vi "Set Calibrator Range.vi"(8 "error in (no error)":errorcluster, 10 "Calibrator Range (0: 10 mV)":u32(ring) items=["10 mV", "25 mV", "100 mV", "250 mV", "1 V", "2.5 V", "Res 50 ohm", "Res 1 Mohm", "Capacitance", "DC", "AC"], 11 "VISA resource name":refnum<visa-resource-name>) -> (0 "error out":errorcluster, 3 "VISA resource name out":refnum<visa-resource-name>)   [LabVIEW 2011, in "Fluke 5XXX Series Multicalibrators.lvlib"]
doc: "This VI programs the instrument range in Pulse, Impedance & Capacitance Measurement and Overload scope modes.\n\nNote:\n\nThis VI is available only for instrument models 5500A and 5520A with oscilloscope option SC600 (SC1100)."
uses:
  Fluke 5XXX Series Multicalibrators.lvlib
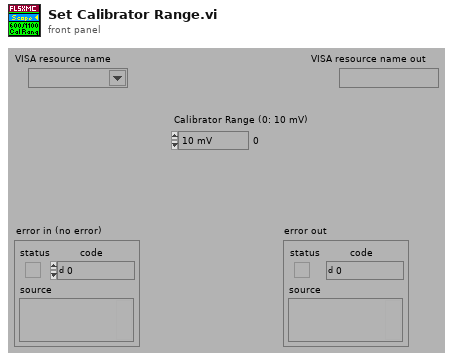
[diagram p1: front panel]
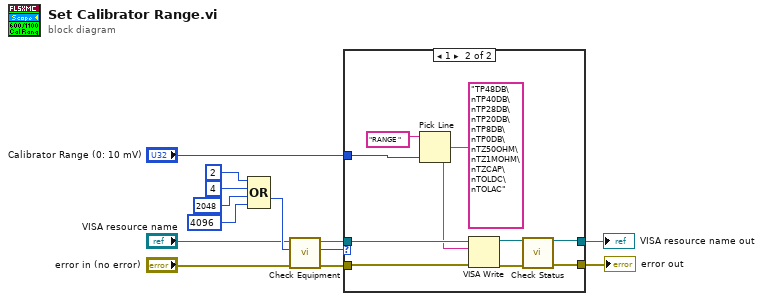
[diagram p0: block diagram]
diagram:
  n1 = Compound Arithmetic op=OR(2 ("Numeric"), 4 ("Numeric"), 2048 ("Numeric"), 4096 ("Numeric")) -> (w8:i32)
  n2 = call "Check Equipment.vi"("error in (no error)"="error in (no error)", "Bit Mask"=w8, "VISA resource name"="VISA resource name") -> ("error out"=w11:errorcluster, "Present?"=w10:u32, "VISA resource name out"=w9:refnum<visa-resource-name>)  [unwired: 6 in]
  n3 = case shown="1" w10 {
    tunnel: [w14 w22] -> w2
    tunnel: w11 -> [w15 w20]
    tunnel: w9 -> [w14 w21]
    tunnel: [w15 w25] -> w3
    tunnel: "Calibrator Range (0: 10 mV)" -> [_ w18]
    frame 0, Default {
    }
    frame 1 {
      n4 = Pick Line(string ("")="RANGE " ("Reset Command"), multi-line string="TP48DB\nTP40DB\nTP28DB\nTP20DB\nTP8DB\nTP0DB\nTZ50OHM\nTZ1MOHM\nTZCAP\nTOLDC\nTOLAC", line index=w18) -> (output string=w17:string)
      n5 = VISA Write(VISA resource name=w21, write buffer=w17, error in (no error)=w20) -> (VISA resource name out=w23:refnum<visa-resource-name>, error out=w24:errorcluster)  [unwired: 1 out]
      n6 = call "Check Status.vi"("VISA resource name"=w23, "error in (no error)"=w24) -> ("VISA resource name out"=w22:refnum<visa-resource-name>, "error out"=w25:errorcluster)  [unwired: 12 in]
    }
  }
  "VISA resource name out" <- w2
  "error out" <- w3
